vi "Set Brake.vi"(8 "error in (no error)":errorcluster, 11 "Dev Elevator in":refnum<class "Dev Elevator.lvclass">) -> (0 "error out":errorcluster, 3 "Dev Elevator out":refnum<class "Dev Elevator.lvclass">)   [LabVIEW 2014, in "Dev Elevator.lvlib" / "Dev Elevator.lvclass"]
uses:
  Dev Elevator.lvclass
  <vilib>/Rock Robotics/WPI/Solenoid/WPI_SolenoidValue.ctl
  Dev Elevator.lvclass/Dev Elevator.ctl
  <vilib>/Rock Robotics/WPI/Solenoid/WPI_SolenoidSetEnum.vi
  Robot/Elevator/Elevator Class/Elevator.lvclass
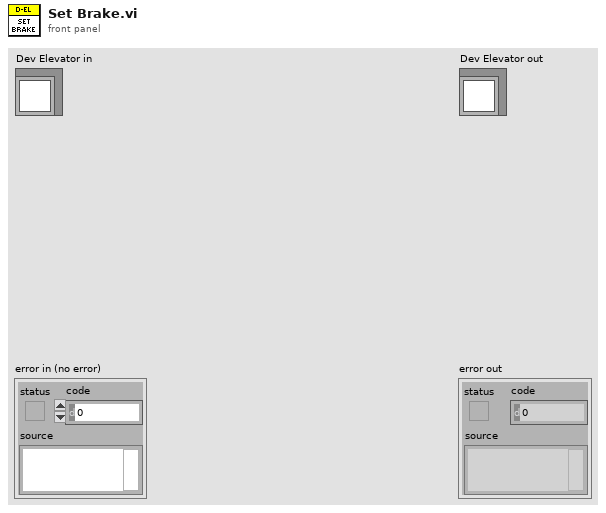
[diagram p1: front panel]
types:
  T1 = typedef "WPI_SolenoidValue.ctl" = enum16{"Off", "On", "Forward", "Reverse"}
  T2 = typedef "WPI_SolenoidDevRef.ctl" = cluster{"DevStatus":errorcluster, "Pneumatics Control Module":u8, "Forward Solenoid Channel":T3, "Reverse Solenoid Channel":T3}
  T3 = typedef "WPI_SolenoidChannel.ctl" = enum8{"Solenoid 0", "Solenoid 1", "Solenoid 2", "Solenoid 3", "Solenoid 4", "Solenoid 5", "Solenoid 6", "Solenoid 7", "Invalid"}
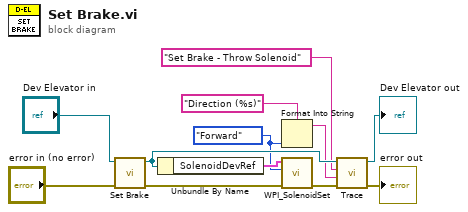
[diagram p0: block diagram]
diagram:
  w2 = WPI_SolenoidValue."Forward" ("Value")
  n1 = call-parent "Set Brake.vi"("error in (no error)"="error in (no error)", "Elevator in"="Dev Elevator in") -> ("error out"=w7:errorcluster, "Elevator out"=w9:refnum<class "Dev Elevator.lvclass">)  [unwired: 8 in]
  n2 = Unbundle By Name(w9) -> ("SolenoidDevRef"=w10:T2)
  n3 = Format Into String(format string="Direction (%s)", w2) -> (resulting string=w1:string)  [unwired: 2 in, 1 out]
  n4 = call-poly <vilib>:"WPI_SolenoidSet.vi"("error in (no error)"=w7, "Value"=w2, "SolenoidDevRef"=w10) -> ("error out"=w6:errorcluster)  [unwired: 7 in, 1 out]
  n5 = call-dynamic "Trace.vi"("error in (no error)"=w6, "System Message"=w1, "System Action"="Set Brake - Throw Solenoid", "System Actor in"=w9) -> ("error out"=→"error out":errorcluster, "System Actor out"=→"Dev Elevator out":refnum<class "Dev Elevator.lvclass">)  [unwired: 6 in]
